vi "decodex_20.vi"() -> ()   [LabVIEW 2021]
panel:
  out "End time":string
  out "Start time":string
  out "array":dbl[][](array[numeric])
  out "Total Time":string
  in  "Stop Button":bool
  out "Total Lines":i32
  out "Total Layers":i32
  out "Z initial":dbl
  in  "Z on/off":bool=TRUE
  in  "Layer height (mm)":dbl=1.0
  in  "file path (use dialog)":path=path "C:/user-Lab/AndreTec/SolidWorks/Teste_4_4_XYS.txt"
  out "Layer":i32
  out "Line":i32
  in  "Velocity (m/s)":dbl=30.0
  in  "Motor - X":refnum<k7>(container)
  in  "Motor - Y":refnum<k7>(container)
  in  "Motor - Z":refnum<k7>(container)
  out "Motor Z":bool=TRUE
  out "Motor X":bool=TRUE
  out "Motor Y":bool=TRUE
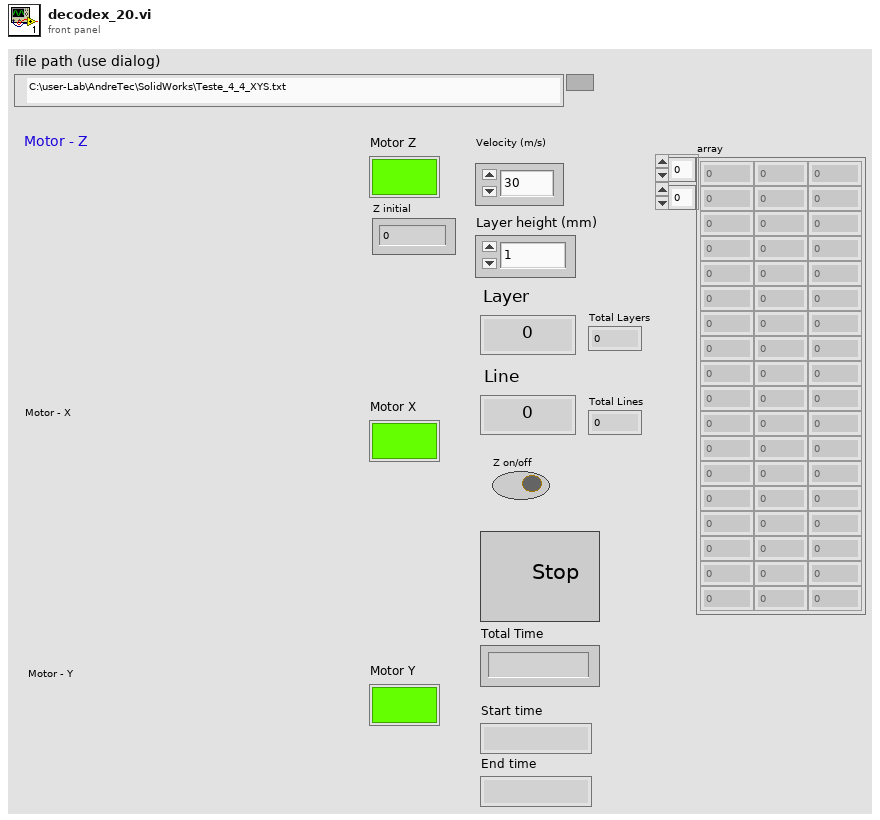
[diagram p1: front panel]
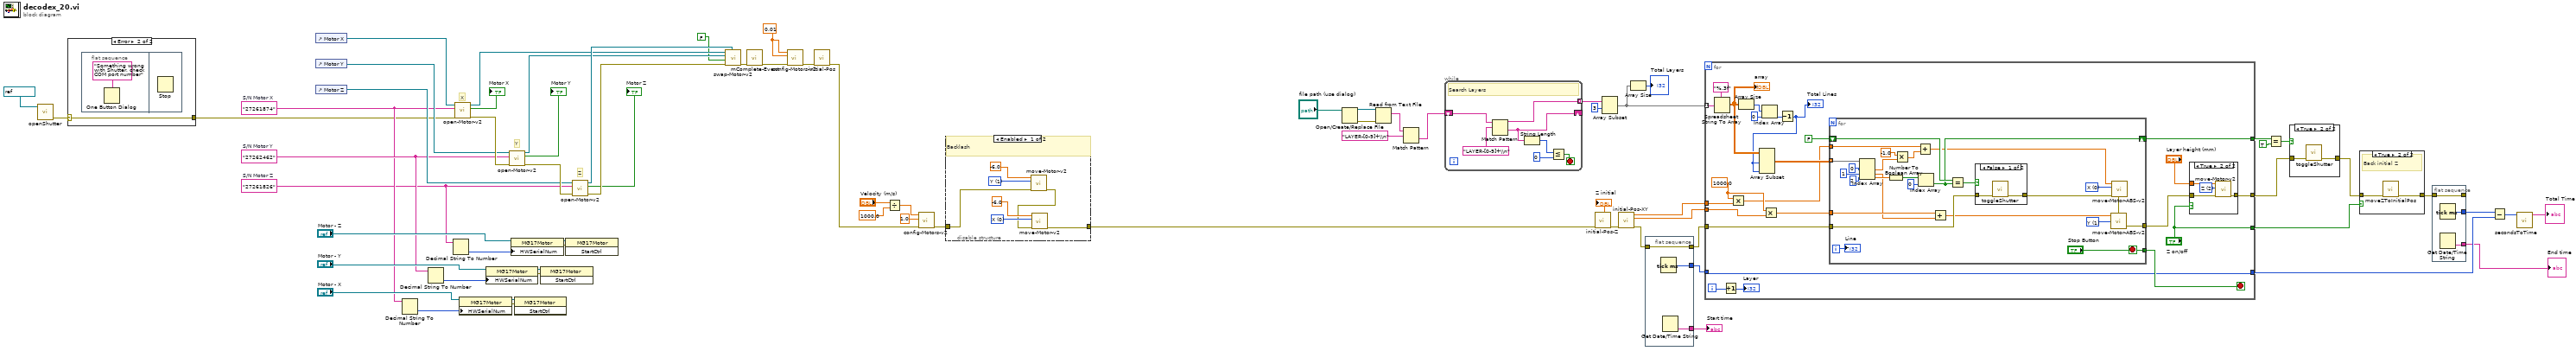
[diagram p0: block diagram]
diagram:
  w61 = 0.01 ("Acc")
  w48 = "27262462"  # S/N Motor Y
  w47 = "27261874"  # S/N Motor X
  w38 = "27261826"  # S/N Motor Z
  # "X"
  # "Y"
  # "Z"
  n1 = call "openShutter.vi"("VISA Refnum in"=refnum<visa-resource-name> "COM3") -> ("error out"=w40:errorcluster)  [unwired: 9 in, 1 out]
  n2 = case shown="Error" w40 {
    selector: w40 -> [w73 w74]
    tunnel: [w73 w74] -> w39
    frame No Error {
    }
    frame Error {
      n3 = flat-sequence {
        frame #0 {
          n4 = One Button Dialog(message="Something wrong with Shutter, check COM port number") -> ()  [unwired: 1 in, 1 out]
        }
        frame #1 {
          n5 = Stop() -> ()  [unwired: 1 in]
        }
      }
    }
  }
  n6 = control-ref of="Motor X"() -> (w69:refnum<vi>)
  n7 = control-ref of="Motor Y"() -> (w68:refnum<vi>)
  n8 = control-ref of="Motor Z"() -> (w64:refnum<vi>)
  n9 = Decimal String To Number(string=w47) -> (number=w49:i32)  [unwired: 2 in, 1 out]
  n10 = Decimal String To Number(string=w48) -> (number=w53:i32)  [unwired: 2 in, 1 out]
  n11 = Decimal String To Number(string=w38) -> (number=w57:i32)  [unwired: 2 in, 1 out]
  n12 = call "open-Motor-v2.vi"("Error In"=w39, "S/N Motor"=w47, "ref Boolean in"=w69) -> ("Error Out"=w72:errorcluster, "Motor Status"=→"Motor X":bool, "Refnum out"=w44:refnum<k7>)  [unwired: 6 in]
  n13 = property class="MG17Motor"(reference="Motor - X", "HWSerialNum"=w49) -> (reference out=w50:refnum<k7>, error out=w51:errorcluster)  [unwired: 1 in]
  n14 = property class="MG17Motor"(reference="Motor - Y", "HWSerialNum"=w53) -> (reference out=w54:refnum<k7>, error out=w55:errorcluster)  [unwired: 1 in]
  n15 = call "open-Motor-v2.vi"("Error In"=w72, "S/N Motor"=w48, "ref Boolean in"=w68) -> ("Error Out"=w66:errorcluster, "Motor Status"=→"Motor Y":bool, "Refnum out"=w43:refnum<k7>)  [unwired: 6 in]
  n16 = property class="MG17Motor"(reference="Motor - Z", "HWSerialNum"=w57) -> (reference out=w58:refnum<k7>, error out=w59:errorcluster)  [unwired: 1 in]
  n17 = invoke class="MG17Motor" method="StartCtrl"(reference=w50, error in=w51) -> ()  [unwired: 1 in, 3 out]
  n18 = invoke class="MG17Motor" method="StartCtrl"(reference=w54, error in=w55) -> ()  [unwired: 1 in, 3 out]
  n19 = invoke class="MG17Motor" method="StartCtrl"(reference=w58, error in=w59) -> ()  [unwired: 1 in, 3 out]
  n20 = call "open-Motor-v2.vi"("Error In"=w66, "S/N Motor"=w38, "ref Boolean in"=w64) -> ("Error Out"=w65:errorcluster, "Motor Status"=→"Motor Z":bool, "Refnum out"=w62:refnum<k7>)  [unwired: 6 in]
  n21 = call "swap-Motor-v2.vi"("Refnum in M3"=w62, "error in (no error)"=w65, "Swap motor"=FALSE, "Refnum in M2"=w43, "Refnum in M1"=w44) -> ("error out"=w46:errorcluster)  [unwired: 6 in]
  n22 = call "mComplete-Event.vi"("Error In"=w46) -> ("Error Out"=w45:errorcluster)  [unwired: 10 in]
  n23 = call "config-Motors-v2.vi"("error in"=w45, "Acc"=w61, "Velocity"=w61) -> ("error out"=w67:errorcluster)  [unwired: 8 in]
  n24 = call "initial-Pos.vi"("error in (no error)"=w67) -> ("error out"=w33:errorcluster)  [unwired: 10 in]
  n25 = Divide(x="Velocity (m/s)", y=1000.0) -> (x/y=w35:dbl)
  n26 = call "config-Motors-v2.vi"("error in"=w33, "Acc"=1.0, "Velocity"=w35) -> ("error out"=w32:errorcluster)  [unwired: 8 in]
  n27 = disable-structure shown="Enabled" {
    disable-tunnel: w32 -> [w78 w83]
    disable-tunnel: [w76 w83] -> w22
    frame Enabled {
      w81 = u16 1 items=["X", "Y", "Z"] ("Axis")
      w82 = u16 0 items=["X", "Y", "Z"] ("Axis")
      # "Backlash"
      n28 = call "move-Motor-v2.vi"("error in"=w78, "Axis"=w81, "Distance (um)"=-6.0) -> ("error out"=w77:errorcluster)  [unwired: 8 in]
      n29 = call "move-Motor-v2.vi"("error in"=w77, "Axis"=w82, "Distance (um)"=-6.0) -> ("error out"=w76:errorcluster)  [unwired: 8 in]
    }
    frame Disabled {
    }
  }
  n30 = Open/Create/Replace File(file path (use dialog)="file path (use dialog)") -> (refnum out=w30:refnum<file>, error out=w31:errorcluster)  [unwired: 5 in, 1 out]
  n31 = Read from Text File(file (use dialog)=w30, error in=w31) -> (text=w29:string)  [unwired: 2 in, 3 out]
  n32 = Match Pattern(string=w29, regular expression="LAYER-[0-9]+\\n") -> (after substring=w27:string)  [unwired: 1 in, 3 out]
  n33 = while {
    shift-right: [w87] -> _
    shift-left: w27 -> [w89]
    tunnel: [w84] -> w26 mode=indexing
    stop <- w85 stop-if-true
    # "Search Layers"
    n34 = Match Pattern(string=w89, regular expression="LAYER-[0-9]+\\n") -> (before substring=w84:string, after substring=w87:string)  [unwired: 1 in, 2 out]
    n35 = String Length(string=w87) -> (length=w88:i32)
    n36 = Less Or Equal?(x=w88, y=0) -> (x <= y?=w85:bool)
  }
  n37 = call "initial-Pos-Z.vi"("error in (no error)"=w22) -> ("error out"=w17:errorcluster, "Z position"=→"Z initial":dbl)  [unwired: 9 in]
  n38 = Array Subset(array=w26, index=3) -> (w19:string[])  [unwired: 1 in]
  n39 = call "initial-Pos-XY.vi"("error in (no error)"=w17) -> ("error out"=w10:errorcluster, "Y position"=w23:dbl, "X position"=w24:dbl)  [unwired: 8 in]
  n40 = Array Size(array=w19) -> (size(s)=→"Total Layers":i32)
  n41 = flat-sequence {
    tunnel: w10 -> [w93]
    tunnel: [w93] -> w9
    tunnel: [w92] -> w7
    tunnel: [w91] -> w2
    frame #0 {
      n42 = Tick Count (ms)() -> (millisecond timer value=w92:u32)
      n43 = Get Date/Time String() -> (time string=w91:string)  [unwired: 3 in, 1 out]
    }
  }
  n44 = for {
    tunnel: w19 -> [w99] mode=indexing
    tunnel: w9 -> [w116]
    tunnel: w24 -> [w104]
    tunnel: w23 -> [w105]
    tunnel: [w111] -> w12
    tunnel: ["Z on/off"] -> w20
    tunnel: [w97] -> w15
    tunnel: w7 -> [w94]
    tunnel: [w94] -> w3
    i -> [w114]
    stop <- w95 stop-if-true
    w103 = 1000.0 ("x")
    n45 = Spreadsheet String To Array(format string="%.3f", spreadsheet string=w99) -> (array=w108:dbl[][])  [unwired: 2 in]
    "array" <- w108
    n46 = Increment(x=w114) -> (x+1=→"Layer":i32)
    n47 = Multiply(x=w103, y=w104) -> (x*y=w102:dbl)
    n48 = Array Size(array=w108) -> (size(s)=w110:i32[])
    n49 = Index Array(array=w110, index=0) -> (element=w107:i32)
    n50 = Multiply(x=w103, y=w105) -> (x*y=w101:dbl)
    n51 = Decrement(x=w107) -> (x-1=w98:i32)
    "Total Lines" <- w98
    n52 = Array Subset(array=w108, length (row)=w98, length (col)=w98) -> (w106:dbl[][])  [unwired: 2 in]
    n53 = for {
      tunnel: w106 -> [w148] mode=indexing
      shift-right: [w127] -> w97
      shift-left: FALSE -> [w141]
      tunnel: w116 -> [w139]
      tunnel: [w134] -> w96
      tunnel: w102 -> [w132]
      tunnel: w101 -> [w131]
      tunnel: ["Stop Button"] -> w95
      i -> [w135]
      stop <- "Stop Button" stop-if-true
      w136 = u16 1 items=["X", "Y", "Z"] ("Axis")
      w137 = u16 0 items=["X", "Y", "Z"] ("Axis")
      n54 = Index Array(array=w148, index #1=0 ("index"), index #2=1 ("index"), index #3=2 ("index")) -> (element #1=w130:dbl, element #2=w129:dbl, element #3=w144:dbl)
      n55 = Number To Boolean Array(number=w144) -> (Boolean array=w143:bool[])
      n56 = Multiply(x=-1.0, y=w130) -> (x*y=w125:dbl)
      n57 = Add(x=w132, y=w125) -> (x+y=w126:dbl)
      n58 = Index Array(array=w143, index=0) -> (element=w127:bool)
      n59 = Add(x=w131, y=w129) -> (x+y=w123:dbl)
      n60 = Equal?(x=w141, y=w127) -> (x = y?=w140:bool)
      n61 = case shown="False" w140 {
        tunnel: w139 -> [w150 w151]
        tunnel: [w149 w151] -> w138
        frame False {
          n62 = call "toggleShutter.vi"("Error In"=w150) -> ("error out"=w149:errorcluster)  [unwired: 9 in]
        }
        frame True {
        }
      }
      n63 = call "move-Motor-ABS-v2.vi"("error in"=w138, "Axis"=w137, "Distance (um)"=w126) -> ("error out"=w133:errorcluster)  [unwired: 8 in]
      n64 = call "move-Motor-ABS-v2.vi"("error in"=w133, "Axis"=w136, "Distance (um)"=w123) -> ("error out"=w134:errorcluster)  [unwired: 8 in]
      "Line" <- w135
    }
    n65 = case shown="True" "Z on/off" {
      tunnel: "Layer height (mm)" -> [_ w121]
      tunnel: [w118 w120] -> w111
      tunnel: w96 -> [w118 w119]
      frame False {
      }
      frame True {
        w122 = u16 2 items=["X", "Y", "Z"] ("Axis")
        n66 = call "move-Motor-v2.vi"("error in"=w119, "Axis"=w122, "Distance (um)"=w121) -> ("error out"=w120:errorcluster)  [unwired: 8 in]
      }
    }
  }
  n67 = Equal?(x=w15, y=TRUE) -> (x = y?=w13:bool)
  n68 = case shown="True" w13 {
    tunnel: w12 -> [w152 w154]
    tunnel: [w152 w153] -> w11
    frame False {
    }
    frame True {
      n69 = call "toggleShutter.vi"("Error In"=w154) -> ("error out"=w153:errorcluster)  [unwired: 9 in]
    }
  }
  n70 = case shown="True" w20 {
    tunnel: [w155 w157] -> w8
    tunnel: w11 -> [w155 w156]
    frame False {
    }
    frame True {
      # "Back initial Z"
      n71 = call "moveZToInitialPos.vi"("error in"=w156) -> ("error out"=w157:errorcluster)  [unwired: 10 in]
    }
  }
  n72 = flat-sequence {
    tunnel: w8 -> [w160]
    tunnel: [w160] -> _
    tunnel: [w159] -> w4
    tunnel: [w158] -> w1
    frame #0 {
      n73 = Tick Count (ms)() -> (millisecond timer value=w159:u32)
      n74 = Get Date/Time String() -> (time string=w158:string)  [unwired: 3 in, 1 out]
    }
  }
  n75 = Subtract(x=w4, y=w3) -> (x-y=w6:u32)
  n76 = call "secondsToTime.vi"("Time input (ms)"=w6) -> ("Time Stamp"=→"Total Time":string)  [unwired: 10 in]
  "Start time" <- w2
  "End time" <- w1
